vi "getCost.vi"(8 "error in (no error)":errorcluster, 11 "Vanilla in":refnum<class "Vanilla.lvclass">) -> (0 "error out":errorcluster, 2 "cost":dbl, 3 "Vanilla out":refnum<class "Vanilla.lvclass">)   [LabVIEW 2018, in "Vanilla.lvclass"]
uses:
  Vanilla.lvclass
  CondimentDecorator/CondimentDecorator.lvclass
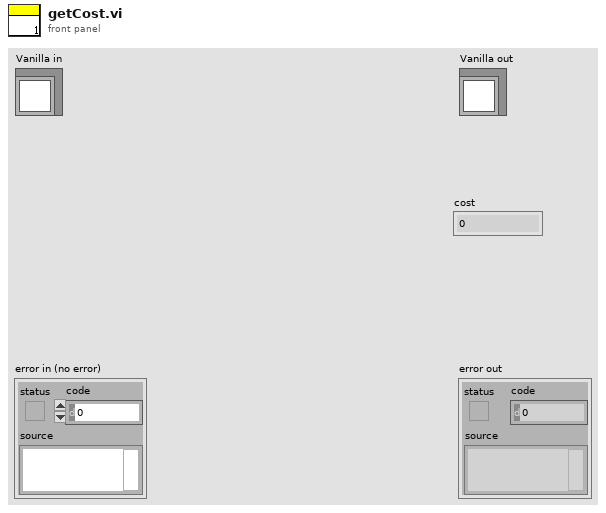
[diagram p1: front panel]
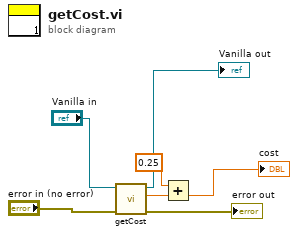
[diagram p0: block diagram]
diagram:
  n1 = call-parent "getCost.vi"("error in (no error)"="error in (no error)", "CondimentDecorator in"="Vanilla in") -> ("error out"=→"error out":errorcluster, "cost"=w6:dbl, "CondimentDecorator out"=→"Vanilla out":refnum<class "Vanilla.lvclass">)  [unwired: 7 in]
  n2 = Add(x=0.25, y=w6) -> (x+y=→"cost":dbl)
